vi "ReplaceEnumWithStringsInClusters.vi"() -> (3 "Flatten XML With Strings":string, 11 "Flatten XML With Enums":string)   [LabVIEW 2020, in "LcWebView.lvclass"]
uses:
  LcWebView.lvclass
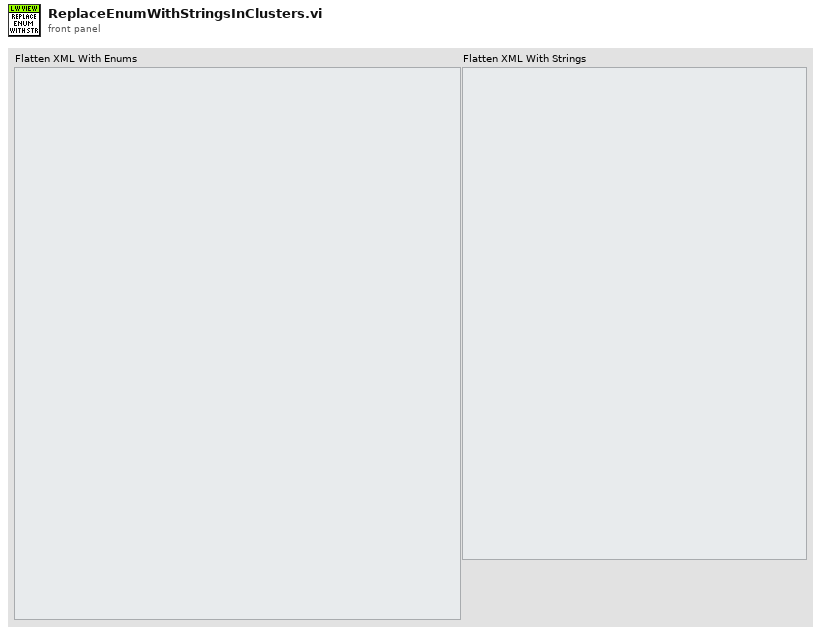
[diagram p1: front panel]
types:
  T1 = cluster{"Text":string, "LegendPosition":enum32{"top", "right", "left", "bottom"}, "LegendPosition":enum16{"top", "right", "left", "bottom"}, "LegendPosition":enum8{"top", "right", "left", "bottom"}, "Number":i32}
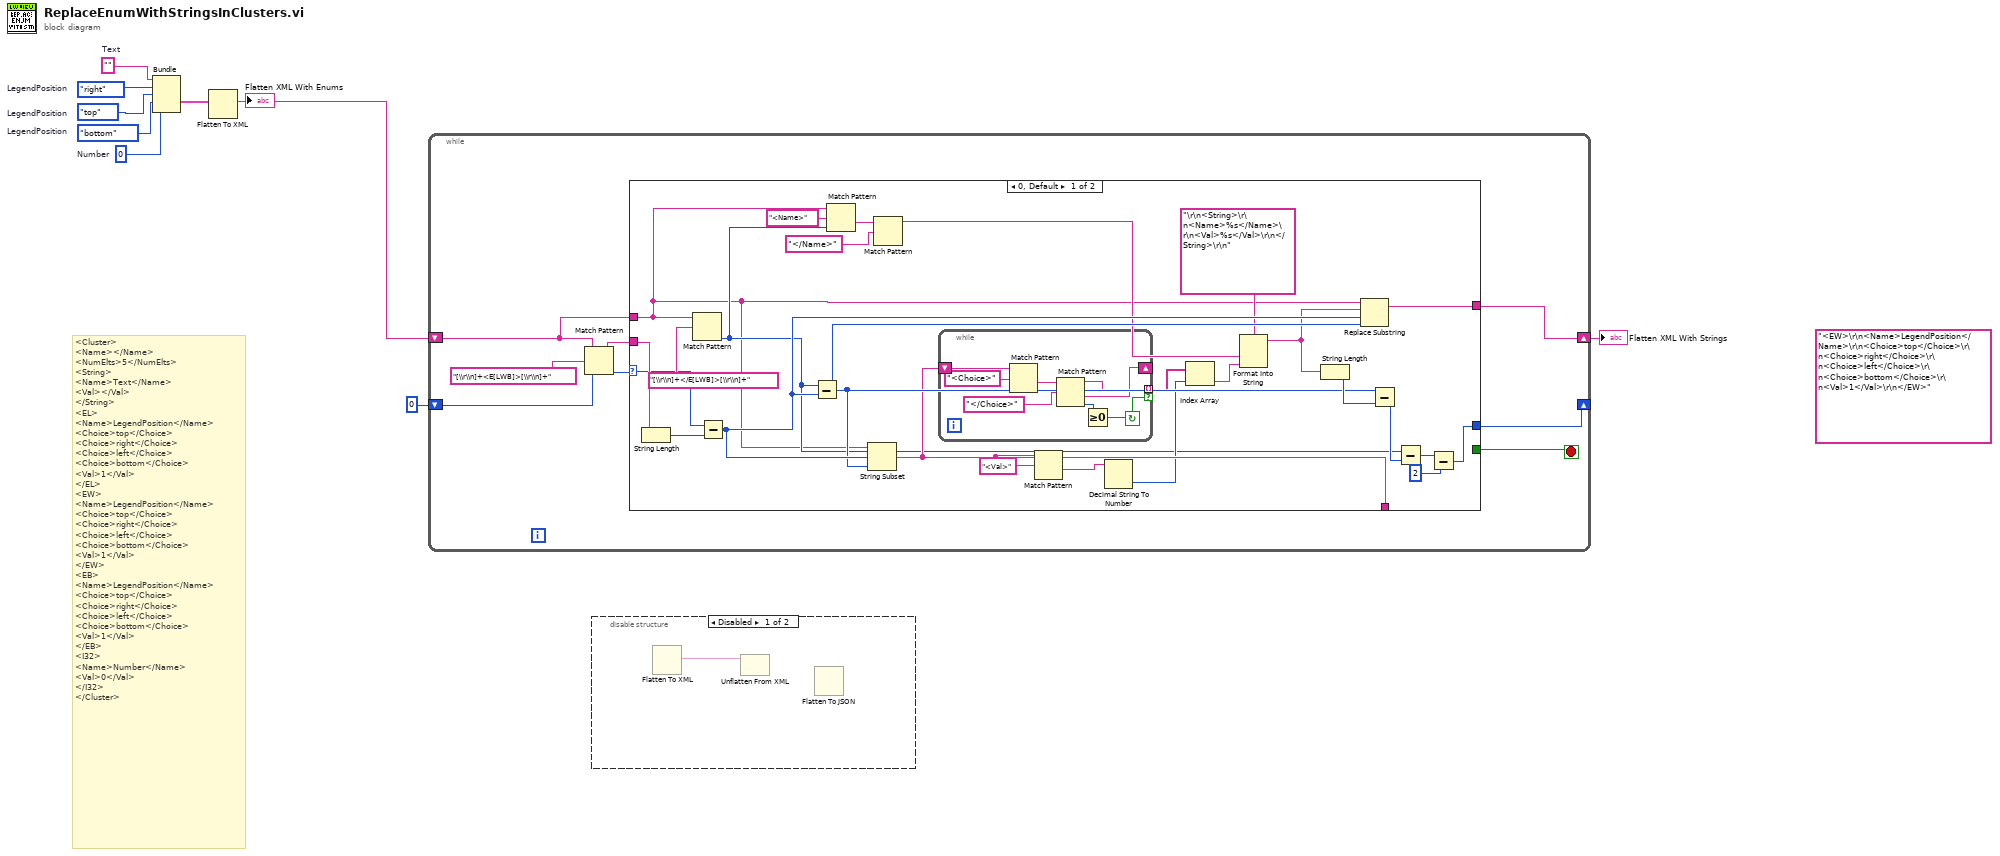
[diagram p0: block diagram]
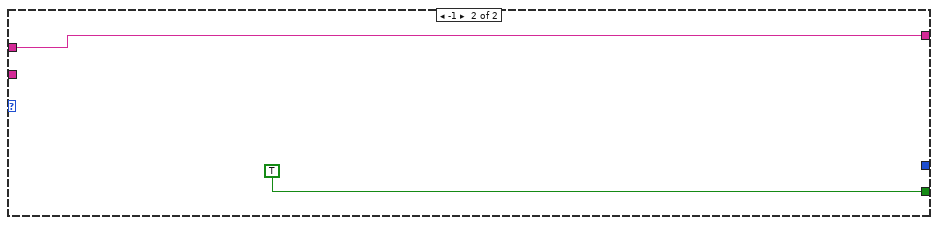
[diagram p3: hidden frame]
diagram:
  w5 = 0  # Number
  w6 = ""  # Text
  w7 = enum8{"top", "right", "left", "bottom"}."bottom"  # LegendPosition
  w8 = enum16{"top", "right", "left", "bottom"}."top"  # LegendPosition
  w9 = enum32{"top", "right", "left", "bottom"}."right"  # LegendPosition
  (unwired) "<EW>\r\n<Name>LegendPosition</Name>\r\n<Choice>top</Choice>\r\n<Choice>right</Choice>\r\n<Choice>left</Choice>\r\n<Choice>bottom</Choice>\r\n<Val>1</Val>\r\n</EW>"
  # "<Cluster>\n<Name></Name>\n<NumElts>5</NumElts>\n<String>\n<Name>Text</Name>\n<Val></Val>\n</String>\n<EL>\n<Name>LegendPosition</Name>\n<Choice>top</Choice>\n<Choice>right</Choice>\n<Choice>left</Choice>\n<Choice>bottom</Choice>\n<Val>1</Val>\n</EL>\n<EW>\n<Name>LegendPosition</Name>\n<Choice>top</Choice>\n<Choice>right</Choice>\n<Choice>left</Choice>\n<Choice>bottom</Choice>\n<Val>1</Val>\n</EW>\n<EB>\n<Name>LegendPosition</Name>\n<Choice>top</Choice>\n<Choice>right</Choice>\n<Choice>left</Choice>\n<Choice>bottom</Choice>\n<Val>1</Val>\n</EB>\n<I32>\n<Name>Number</Name>\n<Val>0</Val>\n</I32>\n</Cluster>"
  n1 = Bundle("Text"=w6, "LegendPosition"=w9, "LegendPosition"=w8, "LegendPosition"=w7, "Number"=w5) -> (w4:T1)  [unwired: 1 in]
  n2 = Flatten To XML(6:w4) -> (2:w3:string)
  "Flatten XML With Enums" <- w3
  n3 = while {
    shift-right: [w11] -> _
    shift-left: 0 -> [w16]
    shift-right: [w10] -> w1
    shift-left: w3 -> [w13]
    stop <- w14 stop-if-true
    n4 = Match Pattern(string=w13, regular expression="[\\r\\n]+<E[LWB]>[\\r\\n]+", offset (0)=w16) -> (match substring=w12:string, offset past match=w15:i32)  [unwired: 2 out]
    n5 = case shown="0, Default" w15 {
      selector: w15 -> [w41 _]
      tunnel: [_ TRUE] -> w14
      tunnel: w13 -> [w21 w52]
      tunnel: w12 -> [w42 _]
      tunnel: [w18 _] -> w11
      tunnel: [w37 w52] -> w10
      tunnel: [w34 _] -> _
      frame 0, Default {
        n6 = String Length(string=w42) -> (length=w40:i32)
        n7 = Match Pattern(string=w21, regular expression="[\\r\\n]+</E[LWB]>[\\r\\n]+") -> (offset past match=w23:i32)  [unwired: 1 in, 3 out]
        n8 = Subtract(x=w41, y=w40) -> (x-y=w36:i32)
        n9 = Subtract(x=w23, y=w36) -> (x-y=w35:i32)
        n10 = Match Pattern(string=w21, regular expression="<Name>", offset (0)=w23) -> (after substring=w25:string)  [unwired: 3 out]
        n11 = String Subset(string=w21, offset (0)=w36, length (rest)=w35) -> (substring=w34:string)
        n12 = Match Pattern(string=w25, regular expression="</Name>") -> (before substring=w22:string)  [unwired: 1 in, 3 out]
        n13 = while {
          shift-right: [w47] -> _
          shift-left: w34 -> [w51]
          tunnel: [w44] -> w31 mode=indexing if=w45
          stop <- w45 continue-if-true
          n14 = Match Pattern(string=w51, regular expression="<Choice>") -> (after substring=w49:string)  [unwired: 1 in, 3 out]
          n15 = Match Pattern(string=w49, regular expression="</Choice>") -> (before substring=w44:string, after substring=w47:string, offset past match=w46:i32)  [unwired: 1 in, 1 out]
          n16 = Greater Or Equal To 0?(x=w46) -> (x >= 0?=w45:bool)
        }
        n17 = Match Pattern(string=w34, regular expression="<Val>") -> (after substring=w32:string)  [unwired: 1 in, 3 out]
        n18 = Decimal String To Number(string=w32) -> (number=w30:i32)  [unwired: 2 in, 1 out]
        n19 = Index Array(array=w31, index=w30) -> (element=w28:string)
        n20 = Format Into String(format string="\r\n<String>\r\n<Name>%s</Name>\r\n<Val>%s</Val>\r\n</String>\r\n", w22, w28) -> (resulting string=w27:string)  [unwired: 2 in, 1 out]
        n21 = String Length(string=w27) -> (length=w39:i32)
        n22 = Replace Substring(2:w35, 3:w36, 4:w27, 5:w21) -> (1:w37:string)  [unwired: 1 out]
        n23 = Subtract(x=w35, y=w39) -> (x-y=w38:i32)
        n24 = Subtract(x=w23, y=w38) -> (x-y=w19:i32)
        n25 = Subtract(x=w19, y=2) -> (x-y=w18:i32)
      }
      frame -1 {
      }
    }
  }
  "Flatten XML With Strings" <- w1
  n26 = disable-structure shown="Disabled" {
    frame Disabled {
      n27 = Flatten To XML() -> (2:w54:string)  [unwired: 1 in]
      n28 = Unflatten From XML(xml string=w54) -> ()  [unwired: 2 in, 2 out]
      n29 = Flatten To JSON() -> ()  [unwired: 3 in, 2 out]
    }
    frame Enabled {
    }
  }
